vi "PH_Tektronix_7000.Fetch Waveform.vi"(0 "i ref in":refnum<vi>, 5 "error IO":errorcluster) -> (14 "i ref out":refnum<vi>, 19 "error out":errorcluster)   [LabVIEW 2014, in "PH_Tektronix_7000.lvlib"]
doc: "If the connection is established, the waveform to fetched is fetched and written to own attributes as well as the errors."
uses:
  PH_Tektronix_7000.lvlib
  instr.lib/Tektronix7000Series/Tektronix 7000 Series - Driver np.lvlib
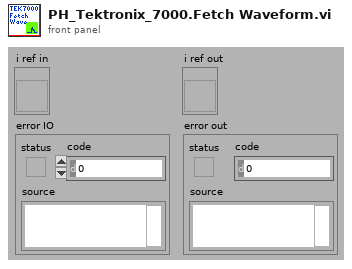
[diagram p1: front panel]
types:
  T1 = typedef "PH_Tektronix_7000.lvlib/PH_Tektronix_7000.i attribute.ctl" = cluster{"VISA Resource Name":refnum<visa-resource-name>, "IDN":cluster{"Instrument Driver":string, "Instrument Firmware":string, "Model":string, "Serial Number":string}, "Selftest":cluster{"Result":i32, "Message":string}, "Trigger Configuration":T2, "Acquisition Configuration":T3, "GUI Refs":T4, "State":T5, "Error Message":string, "Allow Prdc Loop?":bool, "Channel 1":T6, "Channel 2":T6, "Channel 3":T6, "Channel 4":T6, "Data CH 1":waveform(dbl), "Data CH 2":waveform(dbl), "Data CH 3":waveform(dbl), "Data CH 4":waveform(dbl), "Allow config?":bool, "Name Channel 1":string, "Name Channel 2":string, "Name Channel 3":string, "Name Channel 4":string, "Fetch Data before sending to PSDB?":bool, "Constructor passed?":bool, "Data taken at":timestamp, "Plot Colors":u32[], "Default VISA Resource":string}
  T2 = typedef "PH_Tektronix_7000.lvlib/PH_Tektronix_7000.Trigger Config.ctl" = cluster{"Source":u16, "Level [V]":dbl, "Slope":u16, "Coupling":u16, "Trigger Mode":u16}
  T3 = typedef "PH_Tektronix_7000.lvlib/PH_Tektronix_7000.Acquisition Config.ctl" = cluster{"Record Length":u32, "Timebase [s/div]":dbl, "Position [%]":dbl, "Acquisition Type":u16, "Average Waveforms":i32, "Envelope Waveforms":i32, "WfmDB Samples":i32, "Continuous?":bool, "Delay [s]":dbl, "Run?":bool}
  T4 = typedef "PH_Tektronix_7000.lvlib/PH_Tektronix_7000.GUI Refs.ctl" = cluster{"Graph":refnum<vi>, "State":refnum<vi>, "Delete":refnum<vi>, "VISA Resource":refnum<vi>, "Allow Configure":refnum<vi>, "Fetch Data":refnum<vi>, "Fetch before sending Data to PSDB":refnum<vi>, "Name Channel 1":refnum<vi>, "Name Channel 2":refnum<vi>, "Name Channel 3":refnum<vi>, "Name Channel 4":refnum<vi>, "Prdc Intervall [ms]":refnum<vi>, "Data taken":refnum<vi>, "Model":refnum<vi>, "Serial Number":refnum<vi>, "Firmware":refnum<vi>, "Driver":refnum<vi>, "Acquisition":refnum<vi>, "Trigger":refnum<vi>, "Cursor: D Time [s]":refnum<vi>, "Cursor: D Signal [V]":refnum<vi>, "Channel 1":refnum<vi>, "Channel 2":refnum<vi>, "Channel 3":refnum<vi>, "Channel 4":refnum<vi>}
  T5 = typedef "PH_StatusHandler.lvlib/PH_StatusHandler.Status.ctl" = i16
  T6 = typedef "PH_Tektronix_7000.lvlib/PH_Tektronix_7000.Channel Config.ctl" = cluster{"Enable Channel":bool, "Bandwidth":u16, "Input Impedance":u16, "Vertical Coupling":u16, "Probe Attenuation":dbl, "Range [V/div]":dbl, "Position [div]":dbl, "Bandwidth raw":string}
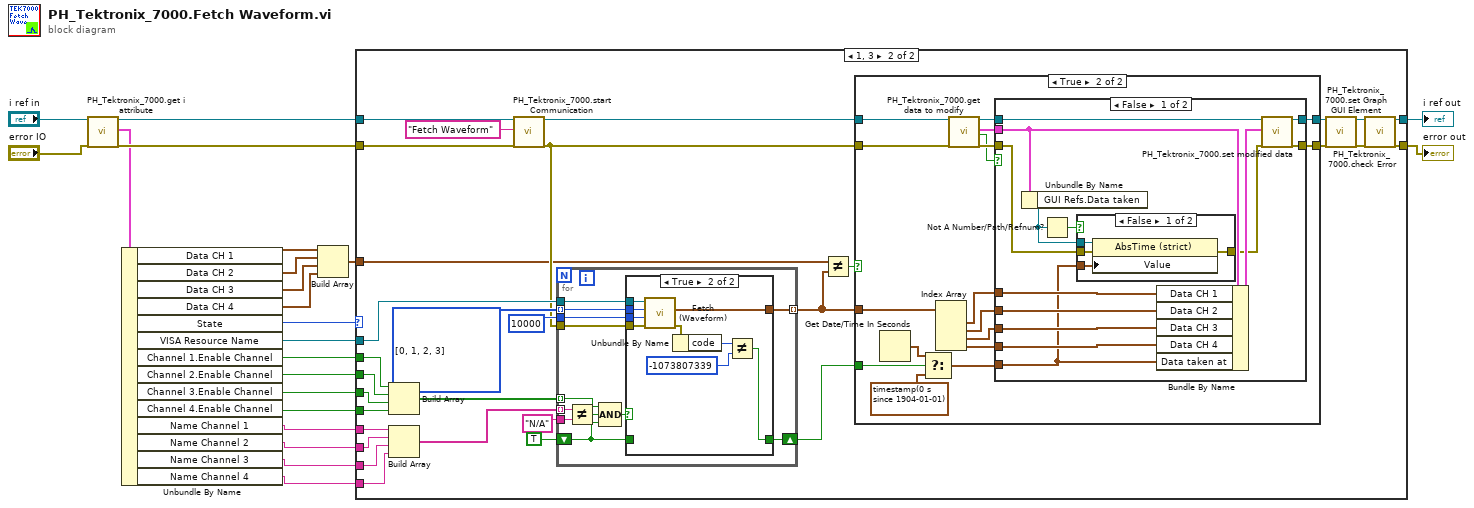
[diagram p0: block diagram]
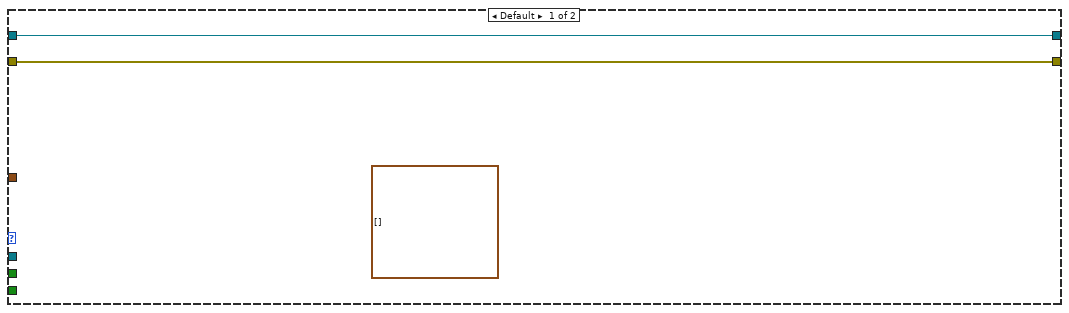
[diagram p2: hidden frame]
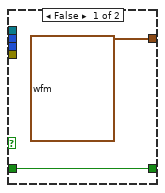
[diagram p6: hidden frame]
diagram:
  n1 = call "PH_Tektronix_7000.get i attribute.vi"("i ref in"="i ref in", "error in (no error)"="error IO") -> ("i ref out"=w18:refnum<vi>, "i attribute"=w20:T1, "error out"=w22:errorcluster)  [unwired: 15 in]
  n2 = Unbundle By Name(w20) -> ("Data CH 1"=w4:waveform(dbl), "Data CH 2"=w3:waveform(dbl), "Data CH 3"=w2:waveform(dbl), "Data CH 4"=w1:waveform(dbl), "State"=w16:T5, "VISA Resource Name"=w21:refnum<visa-resource-name>, "Channel 1.Enable Channel"=w15:bool, "Channel 2.Enable Channel"=w14:bool, "Channel 3.Enable Channel"=w13:bool, "Channel 4.Enable Channel"=w12:bool, "Name Channel 1"=w9:string, "Name Channel 2"=w6:string, "Name Channel 3"=w7:string, "Name Channel 4"=w8:string)
  n3 = Build Array(w4, w3, w2, w1) -> (w5:waveform(dbl)[])
  n4 = case shown="1, 3" w16 {
    tunnel: w18 -> [w24 w41]
    tunnel: w21 -> [_ w43]
    tunnel: [w23 w49] -> w10
    tunnel: w22 -> [w23 w42]
    tunnel: [w24 w50] -> w11
    tunnel: w15 -> [_ w54]
    tunnel: w14 -> [_ w53]
    tunnel: w13 -> [_ w52]
    tunnel: w12 -> [_ w51]
    tunnel: w9 -> [_ w39]
    tunnel: w8 -> [_ w38]
    tunnel: w7 -> [_ w37]
    tunnel: w6 -> [_ w36]
    tunnel: w5 -> [_ w28]
    frame Default {
      (unwired) waveform(dbl)[] []
    }
    frame 1, 3 {
      w48 = u16[] [0, 1, 2, 3] items=["Channel1", "Channel2", "Channel3", "Channel4", "Math1", "Math2", "Math3", "Math3", "Reference1", "Reference2", "Reference3", "Reference4"]
      n5 = Build Array(w54, w53, w52, w51) -> (w46:bool[])
      n6 = Build Array(w39, w36, w37, w38) -> (w35:string[])
      n7 = call "PH_Tektronix_7000.start Communication.vi"("i ref in"=w41, "Action"="Fetch Waveform", "error in"=w42) -> ("i ref out"=w30:refnum<vi>, "error out"=w29:errorcluster)  [unwired: 15 in]
      n8 = for {
        tunnel: w43 -> [w106]
        tunnel: w29 -> [w105]
        tunnel: [w104] -> w31 mode=indexing
        tunnel: w48 -> [w103] mode=indexing
        tunnel: u32 10000 ("Maximum Time (10000ms)") -> [w102]
        tunnel: w46 -> [w99] mode=indexing
        tunnel: w35 -> [w101] mode=indexing
        tunnel: "N/A" -> [w100]
        shift-right: [w96] -> w32
        shift-left: TRUE -> [w95]
        n9 = Not Equal?(x=w101, y=w100) -> (x != y?=w97:bool)
        n10 = Compound Arithmetic op=AND(w99, w97, w95) -> (w98:bool)
        n11 = case shown="True" w98 {
          tunnel: w106 -> [_ w117]
          tunnel: w105 -> [_ w116]
          tunnel: [waveform(dbl) {"t0"=timestamp(0 s since 1904-01-01), "dt"=1.0, "Y"=[]} ("Waveform Data") w115] -> w104
          tunnel: w103 -> [_ w114]
          tunnel: w102 -> [_ w113]
          tunnel: [w107 w109] -> w96
          tunnel: w95 -> [w107 _]
          frame False {
          }
          frame True {
            n12 = call "Fetch (Waveform).vi"("error in (no error)"=w116, "Maximum Time (10000ms)"=w113, "Channel (0:Channel1)"=w114, "VISA resource name"=w117) -> ("error out"=w112:errorcluster, "Waveform Data"=w115:waveform(dbl))  [unwired: 5 in, 1 out]
            n13 = Unbundle By Name(w112) -> ("code"=w111:i32)
            n14 = Not Equal?(x=w111, y=-1073807339) -> (x != y?=w109:bool)
          }
        }
      }
      n15 = Not Equal?(x=w28, y=w31) -> (x != y?=w27:bool)
      n16 = case shown="True" w27 {
        tunnel: [w56 w65] -> w45
        tunnel: [w55 w64] -> w44
        tunnel: w32 -> [_ w63]
        tunnel: w31 -> [_ w59]
        tunnel: w30 -> [w56 w58]
        tunnel: w29 -> [w55 w57]
        frame False {
        }
        frame True {
          n17 = Get Date/Time In Seconds() -> (seconds since 1Jan1904=w62:timestamp)
          n18 = Select(t=w62, s=w63, f=timestamp(0 s since 1904-01-01)) -> (s? t:f=w60:timestamp)
          n19 = Index Array(array=w59) -> (element #1=w69:waveform(dbl), element #2=w68:waveform(dbl), element #3=w67:waveform(dbl), element #4=w66:waveform(dbl))  [unwired: 4 in]
          n20 = call "PH_Tektronix_7000.get data to modify.vi"("i ref in"=w58, "error in (no error)"=w57) -> ("i ref out"=w73:refnum<vi>, "i attribute"=w71:T1, "timed out"=w70:bool, "error out"=w72:errorcluster)  [unwired: 14 in]
          n21 = case shown="False" w70 {
            tunnel: [w87 w93] -> w64
            tunnel: w72 -> [w79 w93]
            tunnel: w73 -> [w86 w94]
            tunnel: [w85 w94] -> w65
            tunnel: w71 -> [w78 _]
            tunnel: w69 -> [w83 _]
            tunnel: w68 -> [w82 _]
            tunnel: w67 -> [w81 _]
            tunnel: w66 -> [w80 _]
            tunnel: w60 -> [w74 _]
            frame False {
              n22 = Unbundle By Name(w78) -> ("GUI Refs.Data taken"=w75:refnum<vi>)
              n23 = Not A Number/Path/Refnum?(number/path/refnum=w75) -> (NaN/Path/Refnum?=w76:bool)
              n24 = case shown="False" w76 {
                tunnel: w79 -> [w91 w92]
                tunnel: [w90 w92] -> w77
                tunnel: w75 -> [w89 _]
                tunnel: w74 -> [w88 _]
                frame False {
                  n25 = property class="AbsTime (strict)"(reference=w89, error in=w91, "Value"=w88) -> (error out=w90:errorcluster)  [unwired: 1 out]
                }
                frame True {
                }
              }
              n26 = Bundle By Name(cluster=w78, "Data CH 1"=w83, "Data CH 2"=w82, "Data CH 3"=w81, "Data CH 4"=w80, "Data taken at"=w74) -> (w84:T1)
              n27 = call "PH_Tektronix_7000.set modified data.vi"("i ref in"=w86, "i attribute"=w84, "error in (no error)"=w77) -> ("i ref out"=w85:refnum<vi>, "error out"=w87:errorcluster)  [unwired: 15 in]
            }
            frame True {
            }
          }
        }
      }
      n28 = call "PH_Tektronix_7000.set Graph GUI Element.vi"("i ref in"=w45, "error in (no error)"=w44) -> ("i ref out"=w26:refnum<vi>, "error out"=w25:errorcluster)  [unwired: 16 in]
      n29 = call "PH_Tektronix_7000.check Error.vi"("i ref in"=w26, "error in"=w25) -> ("i ref out"=w50:refnum<vi>, "error out"=w49:errorcluster)  [unwired: 16 in]
    }
  }
  "i ref out" <- w11
  "error out" <- w10
